vi "ChangeSpecial.vi"() -> ()   [LabVIEW 2020]
uses:
  <vilib>/Utility/config.llb/Write Key (Boolean).vi
  <vilib>/Utility/config.llb/NI_LVConfig.lvlib
panel:
  out "error out":errorcluster
  in  "Radio Buttons":enum32{"Item 0", "Item 1"}(radio)
  in  "SpecialOn":bool
  in  "SpecialOff":bool
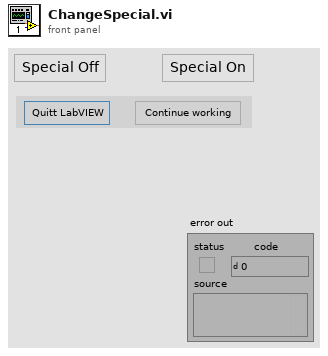
[diagram p1: front panel]
types:
  T1 = typedef "NI_LVConfig.lvlib/Config Data RefNum.ctl" = refnum<k1>
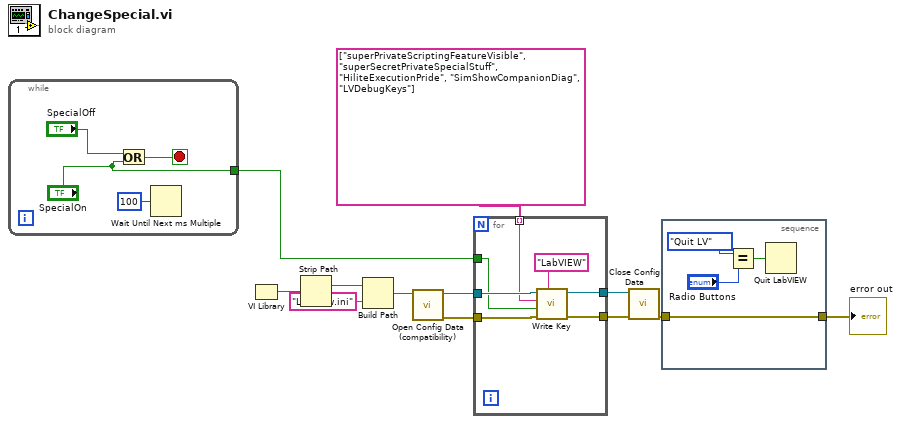
[diagram p0: block diagram]
diagram:
  n1 = while {
    tunnel: ["SpecialOn"] -> w7
    stop <- w15 stop-if-true
    n2 = Or(x="SpecialOff", y="SpecialOn") -> (x .or. y?=w15:bool)
    n3 = Wait Until Next ms Multiple(millisecond multiple=u32 100) -> ()  [unwired: 1 out]
  }
  n4 = VI Library() -> (path=w6:path)
  n5 = Strip Path(path=w6) -> (stripped path=w5:path)  [unwired: 1 out]
  n6 = Build Path(base path=w5, name or relative path="Labview.ini") -> (appended path=w3:path)
  n7 = call <vilib>:"Open Config Data (compatibility).vi"("configuration file path"=w3) -> ("error out"=w12:errorcluster, "refnum"=w9:T1)  [unwired: 8 in, 1 out]
  n8 = for {
    tunnel: w12 -> [w23]
    tunnel: [w22] -> w11
    tunnel: [w21] -> w10
    tunnel: w9 -> [w20]
    tunnel: string[] ["superPrivateScriptingFeatureVisible", "superSecretPrivateSpecialStuff", "HiliteExecutionPride", "SimShowCompanionDiag", "LVDebugKeys"] -> [w18] mode=indexing
    tunnel: w7 -> [w17]
    n9 = call-poly <vilib>:"Write Key.vi"("section"="LabVIEW", "error in (no error)"=w23, "value"=w17, "key"=w18, "refnum"=w20) -> ("error out"=w22:errorcluster, "refnum out"=w21:T1)  [unwired: 4 in, 1 out]
  }
  n10 = call <vilib>:"Close Config Data.vi"("error in (no error)"=w11, "refnum"=w10) -> ("error out"=w1:errorcluster)  [unwired: 8 in, 1 out]
  n11 = stacked-sequence {
    tunnel: [w27] -> w2
    tunnel: w1 -> [w27]
    frame #0 {
      n12 = Equal?(x=enum32{"Quit LV", "Continue\nWorking"}."Quit LV", y="Radio Buttons") -> (x = y?=w26:bool)
      n13 = Quit LabVIEW(quit? (T)=w26) -> ()
    }
  }
  "error out" <- w2
